vi "GetSetAux.vi"(7 "Aux code input":i32, 8 "error in":errorcluster, 9 "Group":T1, 10 "get/set":T2=enum."set", 11 "VISA resource name":refnum<visa-resource-name>) -> (0 "error out":errorcluster, 1 "Aux Decimal Value":i32, 2 "Aux String Value":string, 3 "VISA resource name out":refnum<visa-resource-name>)   [LabVIEW 2023, in "Thermotron 8800.lvlib"]
doc: "AUXE\n\nCommand name: Auxiliaries event status\nCommand type: Variable; edit from hold\nDescription: The query command allows you read the on and off states of the auxiliary groups (1 or 2). Auxiliary group 1 refers to auxiliaries 1-8 and auxiliary group 2 refers to auxiliaries 9-16. The operation command allows you to change the auxiliary states for run manual mode operations and/or edit from hold operations.\nSyntax: \nAUXEn? or AUXEn,ddd\n\nWhere n is an auxiliary group (1 or 2), and where ddd is a three-digit coded integer defined as follows:\n\n1 = AUX 1\n2 = AUX 2\n4 = AUX 3\n8 = AUX 4\n16 = AUX 5\n32 = AUX 6\n64 = AUX 7\n128 = AUX 8\nThe code provides a value between 0 and 255 that adds the values of all the enabled auxiliaries in the selected group. For example, a value of 097 indicates that AUX 7, AUX 6, and AUX 1 are on or turns these auxiliaries on.\nData type: See Syntax.\nQuery example: AUXE1?\n8800 response: 148. (This value indicates that AUX 8, AUX 5, and AUX 3 of auxiliary group 1 are on.)\nOperation example: AUXE1,59\n8800 response: 0 (If the 8800 is in run manual mode, AUX 6, 5, 4, 2, and 1 of auxiliary group 1 are enabled. If they are enabled, the 8800 turns off AUX 8, 7, and 3 of auxiliary group 1.)"
uses:
  Thermotron 8800.lvlib
  Private/get set.ctl
  Private/group.ctl
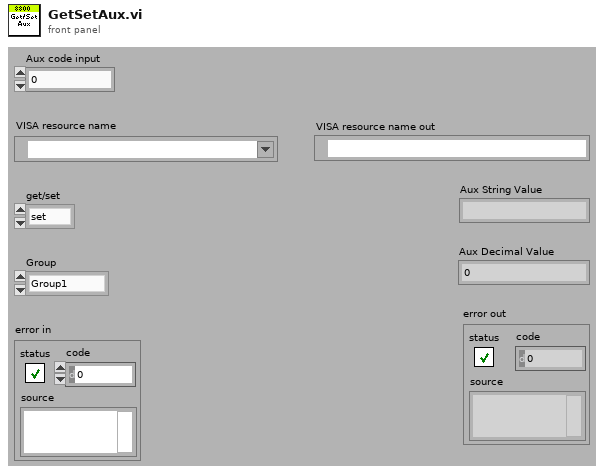
[diagram p1: front panel]
types:
  T1 = typedef "Thermotron 8800.lvlib/group.ctl" = enum16{"Group1", "Group2"}
  T2 = typedef "Thermotron 8800.lvlib/get set.ctl" = enum16{"get", "set"}
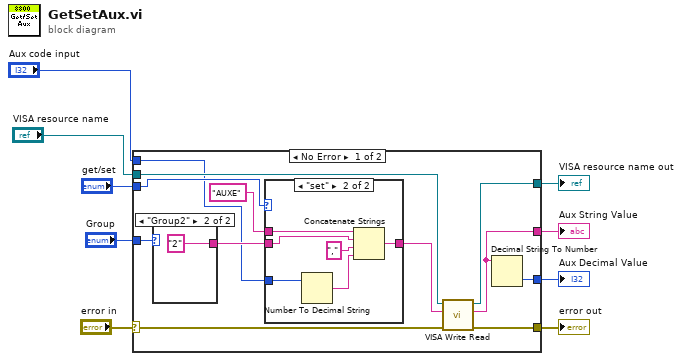
[diagram p0: block diagram]
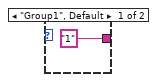
[diagram p2: hidden frame]
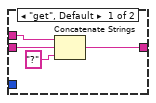
[diagram p3: hidden frame]
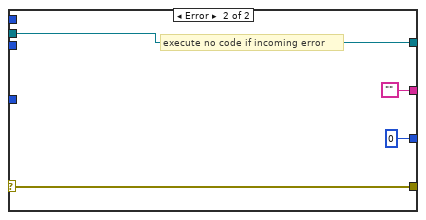
[diagram p4: hidden frame]
diagram:
  n1 = case shown="No Error" "error in" {
    selector: "error in" -> [w10 w36]
    tunnel: [w21 0] -> w9
    tunnel: [w20 ""] -> w8
    tunnel: "VISA resource name" -> [w16 w37]
    tunnel: [w15 w37] -> w6
    tunnel: [w14 w36] -> w5
    tunnel: "get/set" -> [w13 _]
    tunnel: "Group" -> [w12 _]
    tunnel: "Aux code input" -> [w11 _]
    frame No Error {
      n2 = case shown="\"Group2\"" w12 {
        tunnel: ["1" "2"] -> w19
        frame "Group1", Default {
        }
        frame "Group2" {
        }
      }
      n3 = case shown="\"set\"" w13 {
        tunnel: "AUXE" ("8800 Command") -> [w25 w31]
        tunnel: [w26 w29] -> w18
        tunnel: w19 -> [w24 w30]
        tunnel: w11 -> [_ w28]
        frame "get", Default {
          n4 = Concatenate Strings(w25, w24, "?" ("8800 Command")) -> (w26:string)
        }
        frame "set" {
          n5 = Number To Decimal String(number=w28) -> (decimal integer string=w32:string)  [unwired: 1 in]
          n6 = Concatenate Strings(w31, w30, "," ("8800 Command"), w32) -> (w29:string)
        }
      }
      n7 = call "VISA Write Read.vi"("error in (no error)"=w10, "8800 Command"=w18, "VISA Refnum in"=w16) -> ("error out"=w14:errorcluster, "read buffer"=w20:string, "VISA Refnum out"=w15:refnum<visa-resource-name>)  [unwired: 6 in]
      n8 = Decimal String To Number(string=w20) -> (number=w21:i32)  [unwired: 2 in, 1 out]
    }
    frame Error {
      # "execute no code if incoming error"
    }
  }
  "VISA resource name out" <- w6
  "error out" <- w5
  "Aux String Value" <- w8
  "Aux Decimal Value" <- w9
